vi "Vacuum Test - Step 3.vi"(7 "Step":i32, 8 "error in":errorcluster, 9 "Test Results":T9, 10 "Oil In":T1, 11 "Test Configuration":T2) -> (0 "error out":errorcluster, 1 "Test Results Out":T9, 2 "Oil Out":T1, 3 "Test Configuration Out":T2)   [LabVIEW 2015]
uses:
  Controls/Test Results.ctl
  Controls/Step Result.ctl
  Controls/Startup Test.ctl
  Controls/Test Information.ctl
  Controls/Vacuum Test.ctl
  Controls/Test Timing.ctl
  Controls/Vaccum Thresholds.ctl
  Controls/Helium Test.ctl
  Controls/Helium Thresholds.ctl
  Controls/Startup Thresholds.ctl
  CAN Communication/Oil/Typedefs/Session Handle.ctl
  CAN Communication/Oil/Oil.lvclass
panel:
  out "Abs Diff":dbl
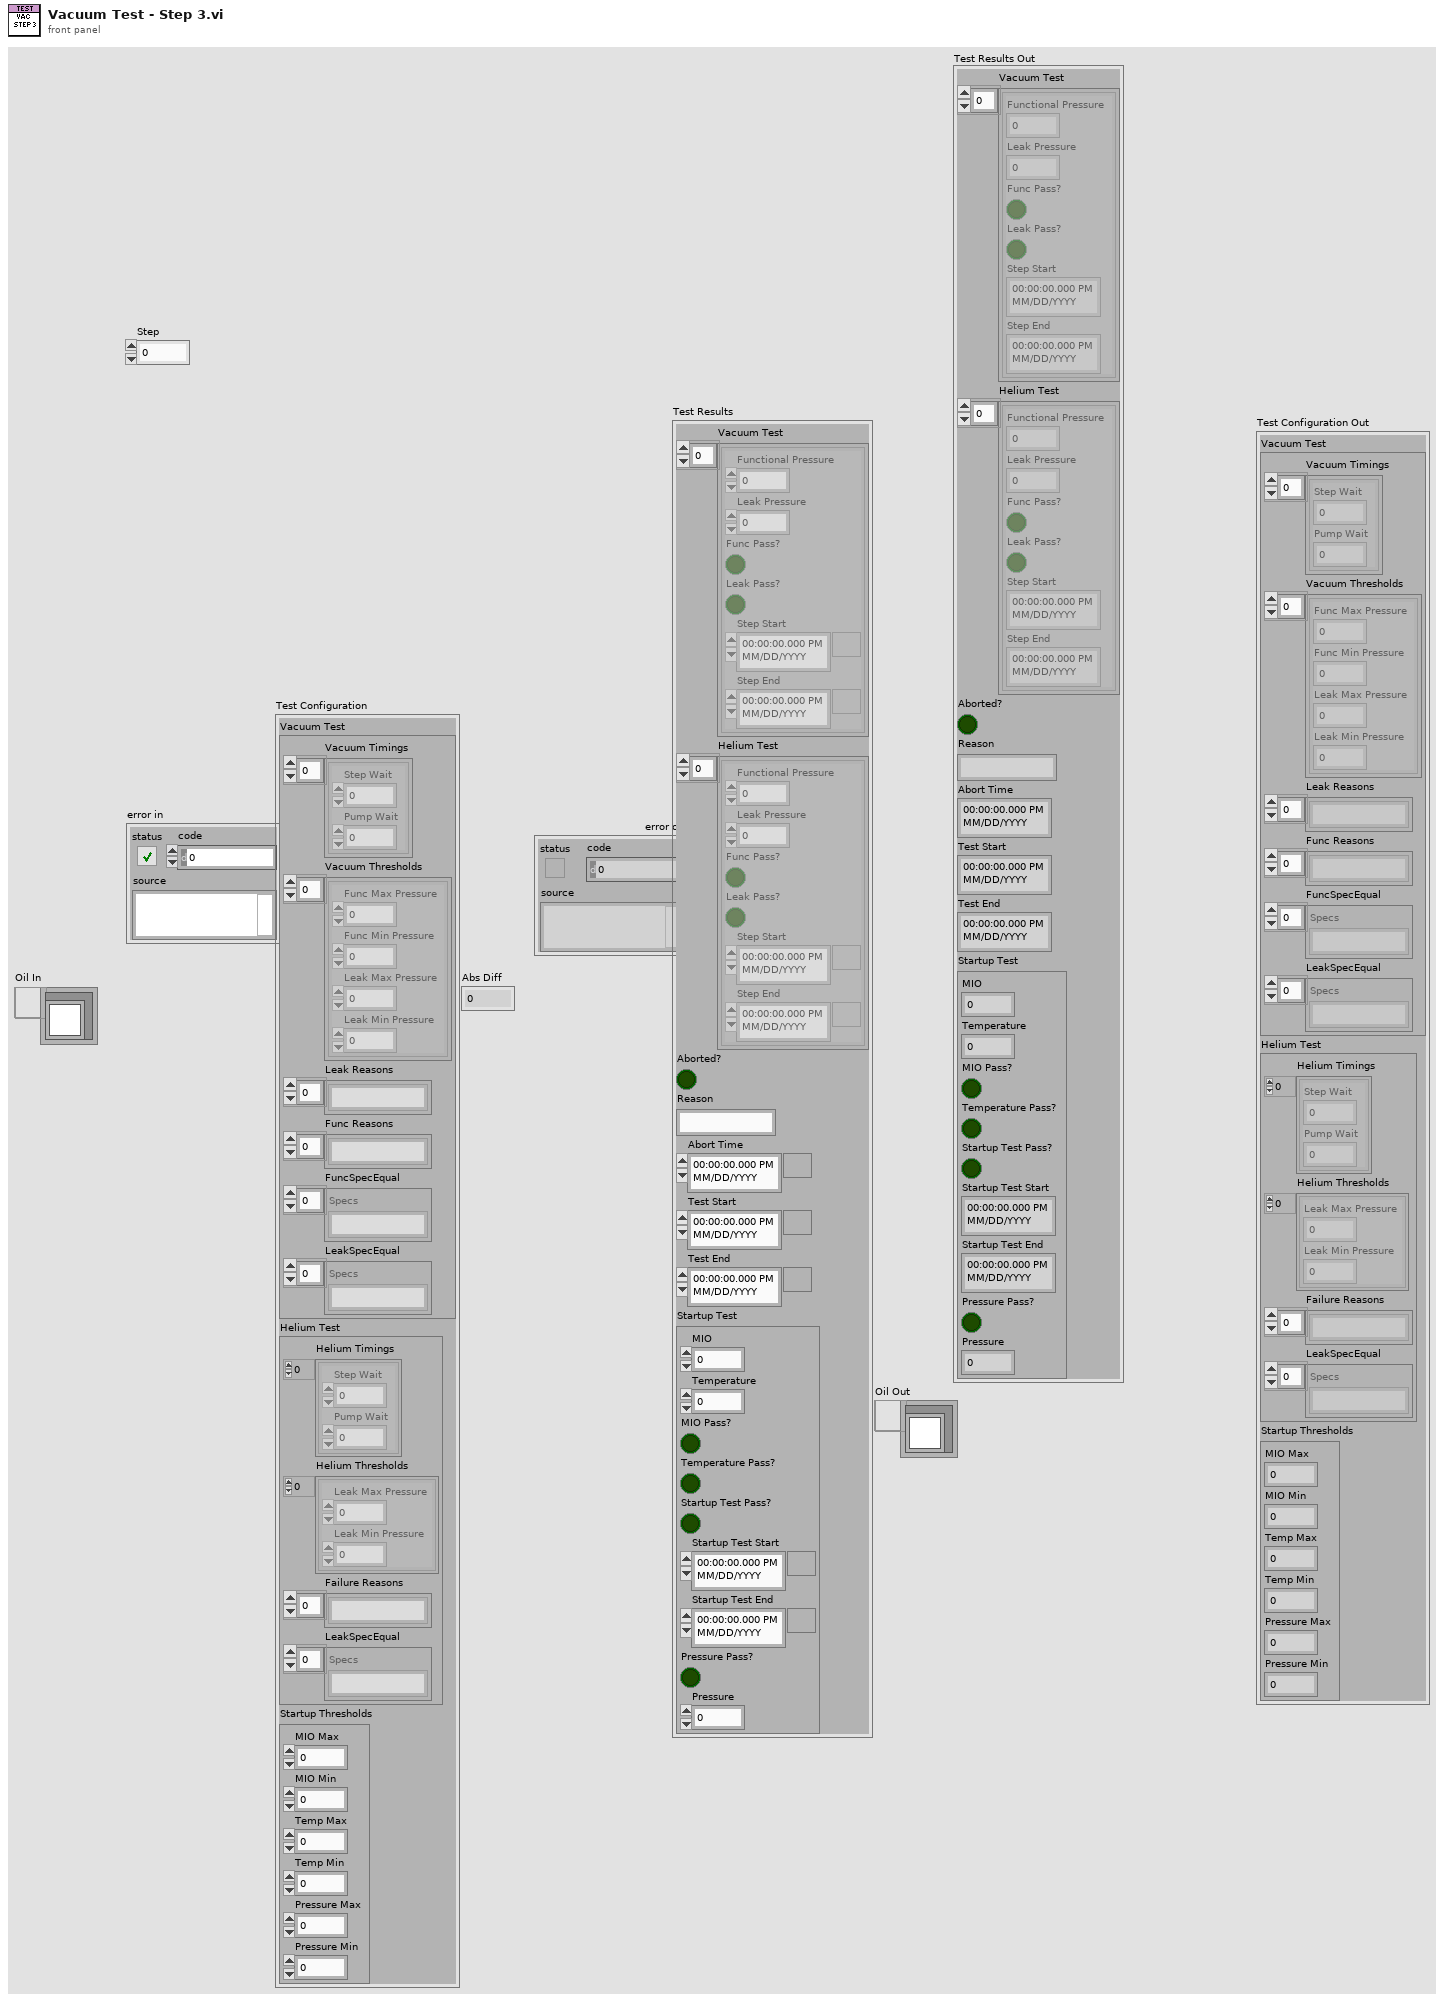
[diagram p1: front panel]
types:
  T1 = typedef "Oil.lvclass/Session Handle.ctl" = refnum<data-value>
  T2 = typedef "Test Information.ctl" = cluster{"Vacuum Test":T3, "Helium Test":T6, "Startup Thresholds":T8}
  T3 = typedef "Vacuum Test.ctl" = cluster{"Vacuum Timings":T4[], "Vacuum Thresholds":T5[], "Leak Reasons":string[], "Func Reasons":string[], "FuncSpecEqual":string[], "LeakSpecEqual":string[]}
  T4 = typedef "Test Timing.ctl" = cluster{"Step Wait":dbl, "Pump Wait":dbl}
  T5 = typedef "Vaccum Thresholds.ctl" = cluster{"Func Max Pressure":dbl, "Func Min Pressure":dbl, "Leak Max Pressure":dbl, "Leak Min Pressure":dbl}
  T6 = typedef "Helium Test.ctl" = cluster{"Helium Timings":T4[], "Helium Thresholds":T7[], "Failure Reasons":string[], "LeakSpecEqual":string[]}
  T7 = typedef "Helium Thresholds.ctl" = cluster{"Leak Max Pressure":dbl, "Leak Min Pressure":dbl}
  T8 = typedef "Startup Thresholds.ctl" = cluster{"MIO Max":dbl, "MIO Min":dbl, "Temp Max":dbl, "Temp Min":dbl, "Pressure Max":dbl, "Pressure Min":dbl}
  T9 = typedef "Test Results.ctl" = cluster{"Vacuum Test":T10[], "Helium Test":T10[], "Aborted?":bool, "Reason":string, "Abort Time":timestamp, "Test Start":timestamp, "Test End":timestamp, "Startup Test":T11}
  T10 = typedef "Step Result.ctl" = cluster{"Functional Pressure":dbl, "Leak Pressure":dbl, "Func Pass?":bool, "Leak Pass?":bool, "Step Start":timestamp, "Step End":timestamp}
  T11 = typedef "Startup Test.ctl" = cluster{"MIO":dbl, "Temperature":dbl, "MIO Pass?":bool, "Temperature Pass?":bool, "Startup Test Pass?":bool, "Startup Test Start":timestamp, "Startup Test End":timestamp, "Pressure Pass?":bool, "Pressure":dbl}
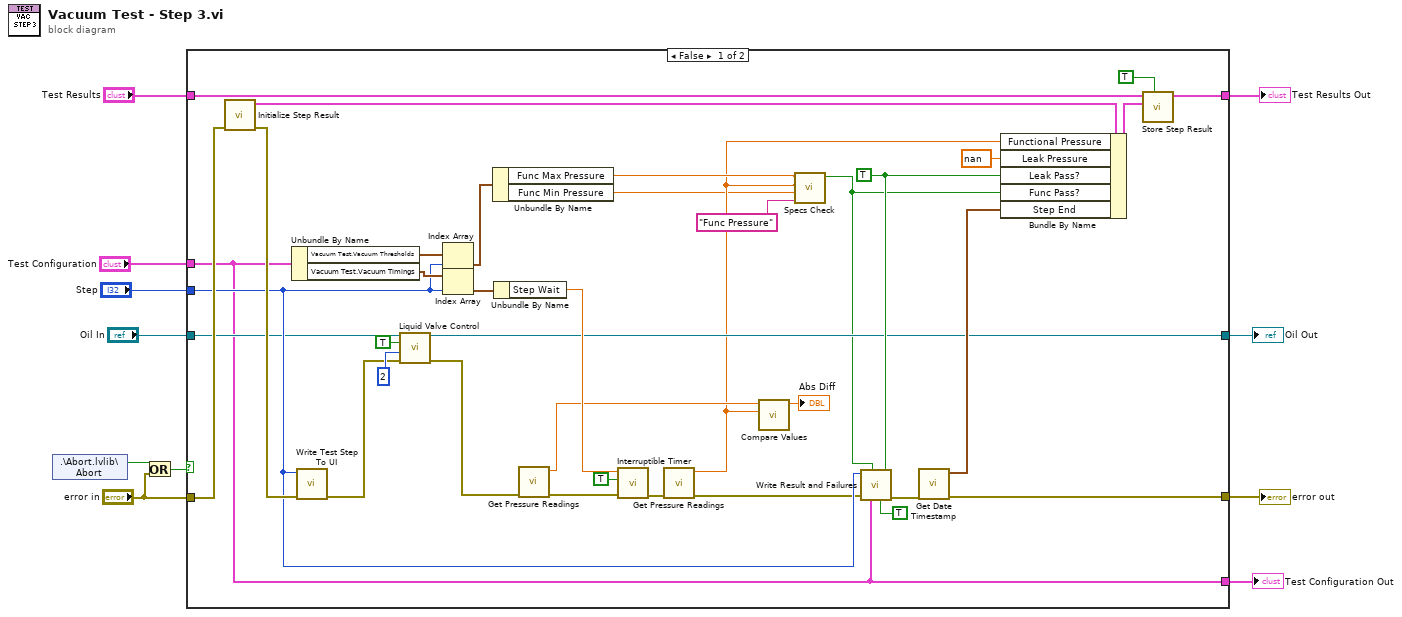
[diagram p0: block diagram]
diagram:
  n1 = shared-variable ".\\Abort.lvlib\\Abort"() -> (w10:bool)  [unwired: 1 in, 1 out]
  n2 = Or(x=w10, y="error in") -> (x .or. y?=w9:bool)
  n3 = case shown="False" w9 {
    tunnel: "error in" -> [w48 w51]
    tunnel: "Test Results" -> [w45 w52]
    tunnel: [w46 w52] -> w8
    tunnel: [w34 w51] -> w7
    tunnel: "Test Configuration" -> [w22 w50]
    tunnel: "Step" -> [w37 _]
    tunnel: [w22 w50] -> w3
    tunnel: [w23 w49] -> w1
    tunnel: "Oil In" -> [w33 w49]
    frame False {
      w24 = TRUE ("Leak Pass?")
      n4 = call "Initialize Step Result.vi"("error in (no error)"=w48) -> ("error out"=w47:errorcluster, "New Step Result"=w44:T10)  [unwired: 8 in, 1 out]
      n5 = Unbundle By Name(w22) -> ("Vacuum Test.Vacuum Thresholds"=w41:T5[], "Vacuum Test.Vacuum Timings"=w40:T4[])
      n6 = call "Write Test Step To UI.vi"("error in (no error)"=w47, "Step"=w37) -> ("error out"=w30:errorcluster)  [unwired: 9 in]
      n7 = call "Liquid Valve Control.vi"("Session Handle in"=w33, "On?"=TRUE, "Valve"=2, "error in (no error)"=w30) -> ("Session Handle out"=w23:T1, "error out"=w20:errorcluster)  [unwired: 8 in, 2 out]
      n8 = Index Array(array=w41, index=w37) -> (element=w38:T5)
      n9 = Index Array(array=w40, index=w37) -> (element=w39:T4)
      n10 = Unbundle By Name(w38) -> ("Func Max Pressure"=w15:dbl, "Func Min Pressure"=w13:dbl)
      n11 = Unbundle By Name(w39) -> ("Step Wait"=w29:dbl)
      n12 = call "Get Pressure Readings.vi"("error in (no error)"=w20) -> ("error out"=w19:errorcluster, "NI-DAQ Pressure"=w18:dbl)  [unwired: 7 in, 2 out]
      n13 = call "Interruptible Timer.vi"("error in (no error)"=w19, "Update UI?"=TRUE, "Wait (s)"=w29) -> ("error out"=w27:errorcluster)  [unwired: 6 in, 2 out]
      n14 = call "Get Pressure Readings.vi"("error in (no error)"=w27) -> ("error out"=w25:errorcluster, "NI-DAQ Pressure"=w14:dbl)  [unwired: 7 in, 2 out]
      n15 = call "Compare Values.vi"("P2"=w14, "P1"=w18) -> ("Abs Diff"=→"Abs Diff":dbl)  [unwired: 9 in]
      n16 = call "Specs Check.vi"("parameter"="Func Pressure", "lower limit"=w13, "x"=w14, "upper limit"=w15) -> ("In Range?"=w16:bool)  [unwired: 6 in, 1 out]
      n17 = call "Write Result and Failures.vi"("Vacuum?"=TRUE, "Leak"=w24, "Test Configuration"=w22, "Func"=w16, "error in (no error)"=w25, "Step"=w37) -> ("error out"=w35:errorcluster)  [unwired: 5 in]
      n18 = call "Get Date Timestamp.vi"("error in (no error)"=w35) -> ("error out"=w34:errorcluster, "current time"=w42:timestamp)  [unwired: 9 in]
      n19 = Bundle By Name(cluster=w44, "Functional Pressure"=w14, "Leak Pressure"=nan, "Leak Pass?"=w24, "Func Pass?"=w16, "Step End"=w42) -> (w43:T10)
      n20 = call "Store Step Result.vi"("Vacuum?"=TRUE, "Step Result"=w43, "Test Results In"=w45) -> ("Test Results Out"=w46:T9)  [unwired: 8 in]
    }
    frame True {
    }
  }
  "error out" <- w7
  "Test Results Out" <- w8
  "Test Configuration Out" <- w3
  "Oil Out" <- w1
